vi "ResetPanes.vi"   [LabVIEW 2012]
uses:
  <vilib>/Utility/miscctls.llb/LVPointTypeDef.ctl
types:
  T1 = typedef "LVPointTypeDef.ctl" = cluster{"Horizontal":i16, "Vertical":i16}
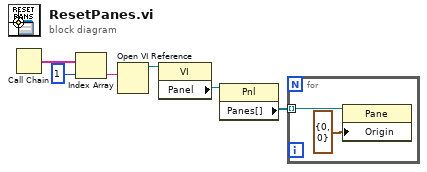
[diagram p0: block diagram]
diagram:
  n1 = Call Chain() -> (call chain=w6:string[])
  n2 = Index Array(array=w6, index=1) -> (element=w4:string)
  n3 = Open VI Reference(vi path=w4) -> (vi reference=w3:refnum<vi>)  [unwired: 5 in, 1 out]
  n4 = property class="VI"(reference=w3) -> ("Panel"=w2:refnum<vi>)  [unwired: 1 in, 2 out]
  n5 = property class="Pnl"(reference=w2) -> ("Panes[]"=w1:refnum<vi>[])  [unwired: 1 in, 2 out]
  n6 = for {
    tunnel: w1 -> [w8] mode=indexing
    n7 = property class="Pane"(reference=w8, "Origin"=T1 {"Horizontal"=0, "Vertical"=0}) -> ()  [unwired: 1 in, 2 out]
  }
